vi "L1WritterReaderIPRTest.vi"() -> ()   [LabVIEW 2012]
panel:
  out "data read value":u32
  out "IPR_Data":string="0_2-0@0\r\n"
  out "Reg 65":string="0_2-0@0\r\n"
  in  "Address 2":i32=70
  out "Data READ":string="empty_read_buffer"
  out "error out":errorcluster
  in  "error in (no error)":errorcluster
  in  "Data":i32=65
  in  "Address":i32
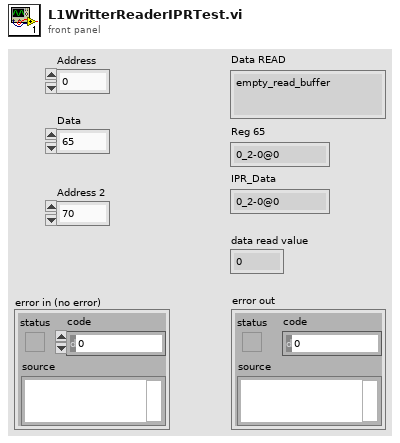
[diagram p1: front panel]
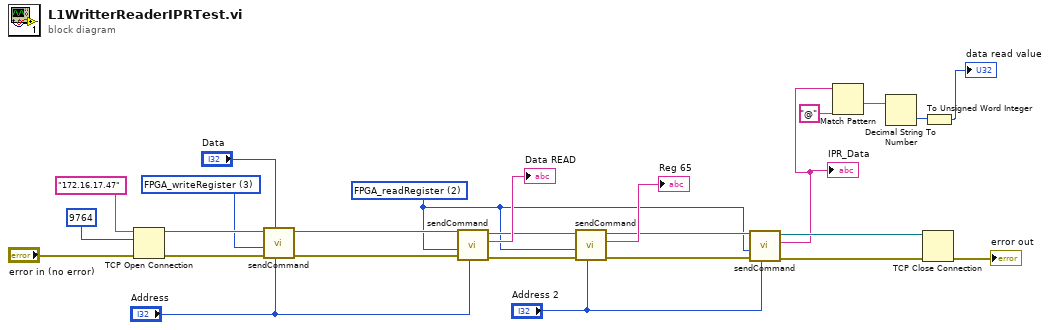
[diagram p0: block diagram]
diagram:
  w8 = u16 2 items=["sendCommand"=9, "FPGA_writeRegister"=3, "FPGA_readRegister"=2, "uC_writeRegister"=1, "uC_readRegister"=0] ("Action")
  w19 = u16 3 items=["sendCommand"=9, "FPGA_writeRegister"=3, "FPGA_readRegister"=2, "uC_writeRegister"=1, "uC_readRegister"=0] ("Action")
  n1 = TCP Open Connection(address="172.16.17.47", remote port or service name=9764, error in (no error)="error in (no error)") -> (connection ID=w20:refnum<k5>, error out=w21:errorcluster)  [unwired: 2 in]
  n2 = call "sendCommand.vi"("Address"="Address", "Data"="Data", "error in"=w21, "Action"=w19, "connection ID"=w20) -> ("error out"=w18:errorcluster, "connection ID out"=w17:refnum<k5>)  [unwired: 2 in, 3 out]
  n3 = call "sendCommand.vi"("Address"="Address", "error in"=w18, "Action"=w8, "connection ID"=w17) -> ("error out"=w13:errorcluster, "Data out"=→"Data READ":string, "connection ID out"=w15:refnum<k5>)  [unwired: 3 in, 2 out]
  n4 = call "sendCommand.vi"("Address"="Address 2", "error in"=w13, "Action"=w8, "connection ID"=w15) -> ("error out"=w12:errorcluster, "Data out"=→"Reg 65":string, "connection ID out"=w11:refnum<k5>)  [unwired: 3 in, 2 out]
  n5 = call "sendCommand.vi"("Address"="Address 2", "error in"=w12, "Action"=w8, "connection ID"=w11) -> ("error out"=w9:errorcluster, "Data out"=w1:string, "connection ID out"=w10:refnum<k5>)  [unwired: 3 in, 2 out]
  "IPR_Data" <- w1
  n6 = Match Pattern(string=w1, regular expression="@" ("search string/char (-)")) -> (after substring=w4:string)  [unwired: 1 in, 3 out]
  n7 = Decimal String To Number(string=w4) -> (number=w3:i32)  [unwired: 2 in, 1 out]
  n8 = TCP Close Connection(connection ID=w10, error in (no error)=w9) -> (error out=→"error out":errorcluster)  [unwired: 1 in, 1 out]
  n9 = To Unsigned Word Integer(number=w3) -> (unsigned 16bit integer=→"data read value":u16)
